vi "TOF TOGGLE.vi"(9 "Delay (ms)":u32=500, 10 "Input":bool) -> (2 "Output":bool)   [LabVIEW 2015]
doc: "Similar to a toggle, with a TOF timer built in.\nThe TOF TOGGLE, when given a True input, will immediately output true. When the input reverts back to False, the output will wait for the specified delay to elapse before outputting False.\n\nIf the Delay is set to 0, this will simply act as a toggle."
panel:
  in  "Delay_TOF":T1={"Timer_States"=enum."Input_True", "Delay-Done_Time"=0, "Toggle-State"=enum."Button-False", "Toggle Last"=FALSE}
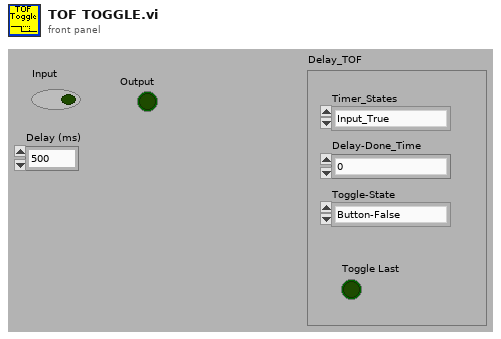
[diagram p1: front panel]
types:
  T1 = cluster{"Timer_States":enum16{"Input_True", "Input_False_Timing", "Input_False_Timing_Complete"}, "Delay-Done_Time":u32, "Toggle-State":enum16{"Button True-Waiting", "Button-False"}, "Toggle Last":bool}
  T2 = enum16{"Input_True", "Input_False_Timing", "Input_False_Timing_Complete"}
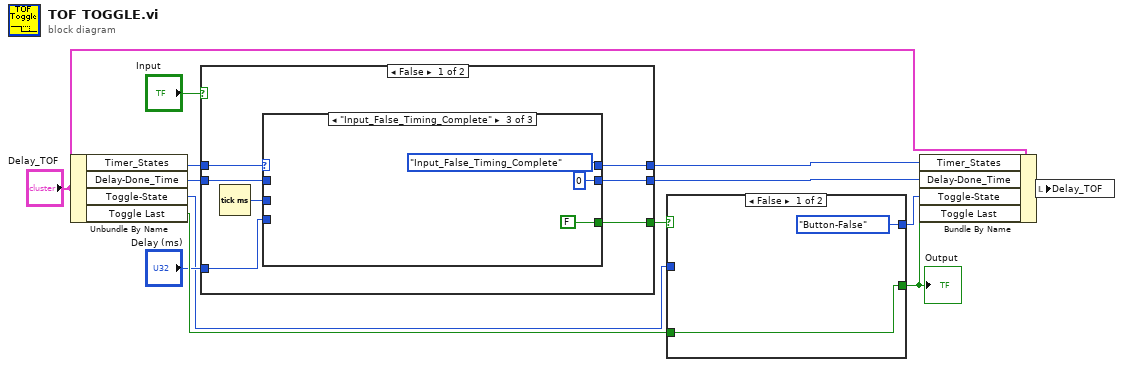
[diagram p0: block diagram]
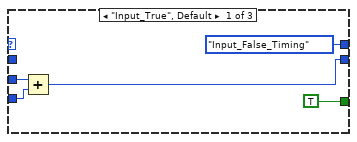
[diagram p2: hidden frame]
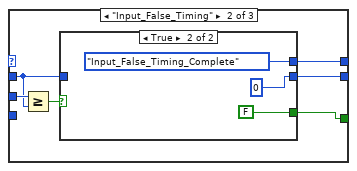
[diagram p3: hidden frame]
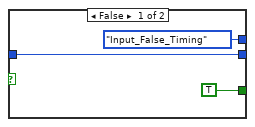
[diagram p4: hidden frame]
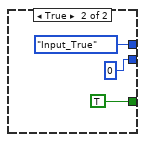
[diagram p5: hidden frame]
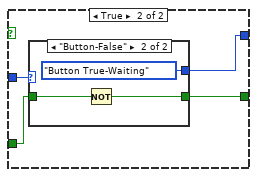
[diagram p6: hidden frame]
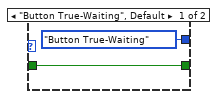
[diagram p7: hidden frame]
diagram:
  n1 = Unbundle By Name("Delay_TOF") -> ("Timer_States"=w6:T2, "Delay-Done_Time"=w4:u32, "Toggle-State"=w3:enum16{"Button True-Waiting", "Button-False"}, "Toggle Last"=w11:bool)
  n2 = case shown="False" "Input" {
    tunnel: [w17 TRUE] -> w8
    tunnel: [w18 T2."Input_True" ("Timer_States")] -> w1
    tunnel: [w19 u32 0 ("Delay-Done_Time")] -> w2
    tunnel: w6 -> [w16 _]
    tunnel: "Delay (ms)" -> [w15 _]
    tunnel: w4 -> [w14 _]
    frame False {
      n3 = Tick Count (ms)() -> (millisecond timer value=w20:u32)
      n4 = case shown="\"Input_False_Timing_Complete\"" w16 {
        tunnel: w20 -> [w24 w31 _]
        tunnel: [w23 w27 u32 0 ("Delay-Done_Time")] -> w19
        tunnel: [T2."Input_False_Timing" ("Timer_States") w29 T2."Input_False_Timing_Complete" ("Timer_States")] -> w18
        tunnel: [TRUE w28 FALSE] -> w17
        tunnel: w15 -> [w21 _ _]
        tunnel: w14 -> [_ w26 _]
        frame "Input_True", Default {
          n5 = Add(x=w24, y=w21) -> (x+y=w23:u32)
        }
        frame "Input_False_Timing" {
          n6 = Greater Or Equal?(x=w31, y=w26) -> (x >= y?=w30:bool)
          n7 = case shown="True" w30 {
            tunnel: [T2."Input_False_Timing" ("Timer_States") T2."Input_False_Timing_Complete" ("Timer_States")] -> w29
            tunnel: [TRUE FALSE] -> w28
            tunnel: [w32 u32 0 ("Delay-Done_Time")] -> w27
            tunnel: w26 -> [w32 _]
            frame False {
            }
            frame True {
            }
          }
        }
        frame "Input_False_Timing_Complete" {
        }
      }
    }
    frame True {
    }
  }
  n8 = case shown="False" w8 {
    tunnel: [w45 w48] -> w9
    tunnel: w11 -> [w45 w49]
    tunnel: [enum16{"Button True-Waiting", "Button-False"}."Button-False" ("Toggle-State") w47] -> w10
    tunnel: w3 -> [_ w46]
    frame False {
    }
    frame True {
      n9 = case shown="\"Button-False\"" w46 {
        tunnel: w49 -> [w51 w54]
        tunnel: [w51 w53] -> w48
        tunnel: [enum16{"Button True-Waiting", "Button-False"}."Button True-Waiting" ("Toggle-State") enum16{"Button True-Waiting", "Button-False"}."Button True-Waiting" ("Toggle-State")] -> w47
        frame "Button True-Waiting", Default {
        }
        frame "Button-False" {
          n10 = Not(x=w54) -> (.not. x?=w53:bool)
        }
      }
    }
  }
  "Output" <- w9
  n11 = Bundle By Name(cluster="Delay_TOF", "Timer_States"=w1, "Delay-Done_Time"=w2, "Toggle-State"=w10, "Toggle Last"=w9) -> (w12:T1)
  n12 = local write "Delay_TOF"(w12) -> ()
